vi "CIF_CIPC Channel Performance Test.vi"() -> ()   [LabVIEW 2021]
uses:
  <vilib>/Platform/TimedLoop/XDataNode/XDataNode.xnode
  <vilib>/Platform/TimedLoop/XDataNode/nitl_modes.ctl
  <vilib>/Platform/TimedLoop/XDataNode/XDNodeRunTimeDep.lvlib
  <vilib>/Platform/TimedLoop/XDataNode/wakeup.ctl
  <vilib>/Platform/TimedLoop/XDataNode/timing_clust.ctl
  CIFChannels/Typedef/Direction.ctl
  CIFChannels/CIFChannels.lvclass
  Double/CIF_CIPC_Chn_Double.lvclass
  826832b0-dd6f-429a-ad13-ef368b1fb745.vi
  9775e11d-bb16-4108-996d-a0b506d5c84d.vi
  c8328e1c-7f53-4066-9f95-efcf565d42f9.vi
  <vilib>/CIF Foundation/CIF CIPC/CIF_NI_CIPC.lvlib
  44731855-fec1-40f2-bc70-5f443bf403a0.vi
  ChannelCommon/typedef/New FIFO Instance Response.ctl
  ChannelCommon/ChannelCommon.lvlib
panel:
  in  "Stop":bool
  out "avg dbl channel":dbl
  out "max dbl channel":dbl
  out "avg raw channel":dbl
  out "max raw channel":dbl
  out "pass":bool
  out "error out":errorcluster
  # "This test should be run on RT.  It stresses the communications by constantly creating resource contraints with the low priority sender and the high priority loop. On Windows the priority of the loops cannot be set."
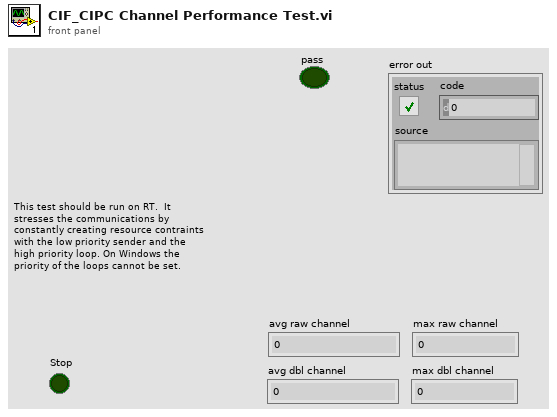
[diagram p1: front panel]
types:
  T1 = typedef "XDNodeRunTimeDep.lvlib/timing_clust.ctl" = cluster{"Expected End [f-1]":u64, "Actual End [f-1]":u64, "Finished Late? [f-1]":bool, "Expected End [i-1]":u64, "Actual End [i-1]":u64, "Finished Late? [i-1]":bool, "Expected Start [i]":u64, "Actual Start [i]":u64, "Expected Start [f]":u64, "Actual Start [f]":u64, "Source Name":string, "Structure Name":string, "Period":i64, "Deadline":i64, "Offset":i64, "Start":i64, "Priority":i32, "Timeout":i32, "Mode":T2, "Wakeup Reason":T3, "Error":errorcluster, "Source Type":string, "Secondary Source Type":string, "Global End Time":u64, "Global Start Time":u64, "Frame Duration":u64, "Iteration Duration":u64, "Assigned CPU":i32, "I/O Scan Engine Mode":u32}
  T2 = typedef "XDNodeRunTimeDep.lvlib/nitl_modes.ctl" = enum32{"No Change", "Process missed periods, maintain original phase", "Discard missed periods, maintain original phase", "Process missed periods, ignore original phase", "Discard missed periods, ignore original phase"}
  T3 = typedef "XDNodeRunTimeDep.lvlib/wakeup.ctl" = enum32{"Normal", "Aborted", "Asynchronous wakeup", "Timing source error", "Timed loop error", "Timeout"}
  T4 = typedef "ChannelCommon.lvlib/New FIFO Instance Response.ctl" = cluster{"Publisher":string, "Custom Data":u8[]}
  T5 = typedef "CIFChannels.lvclass/Direction.ctl" = enum16{"Publisher", "Subscriber"}
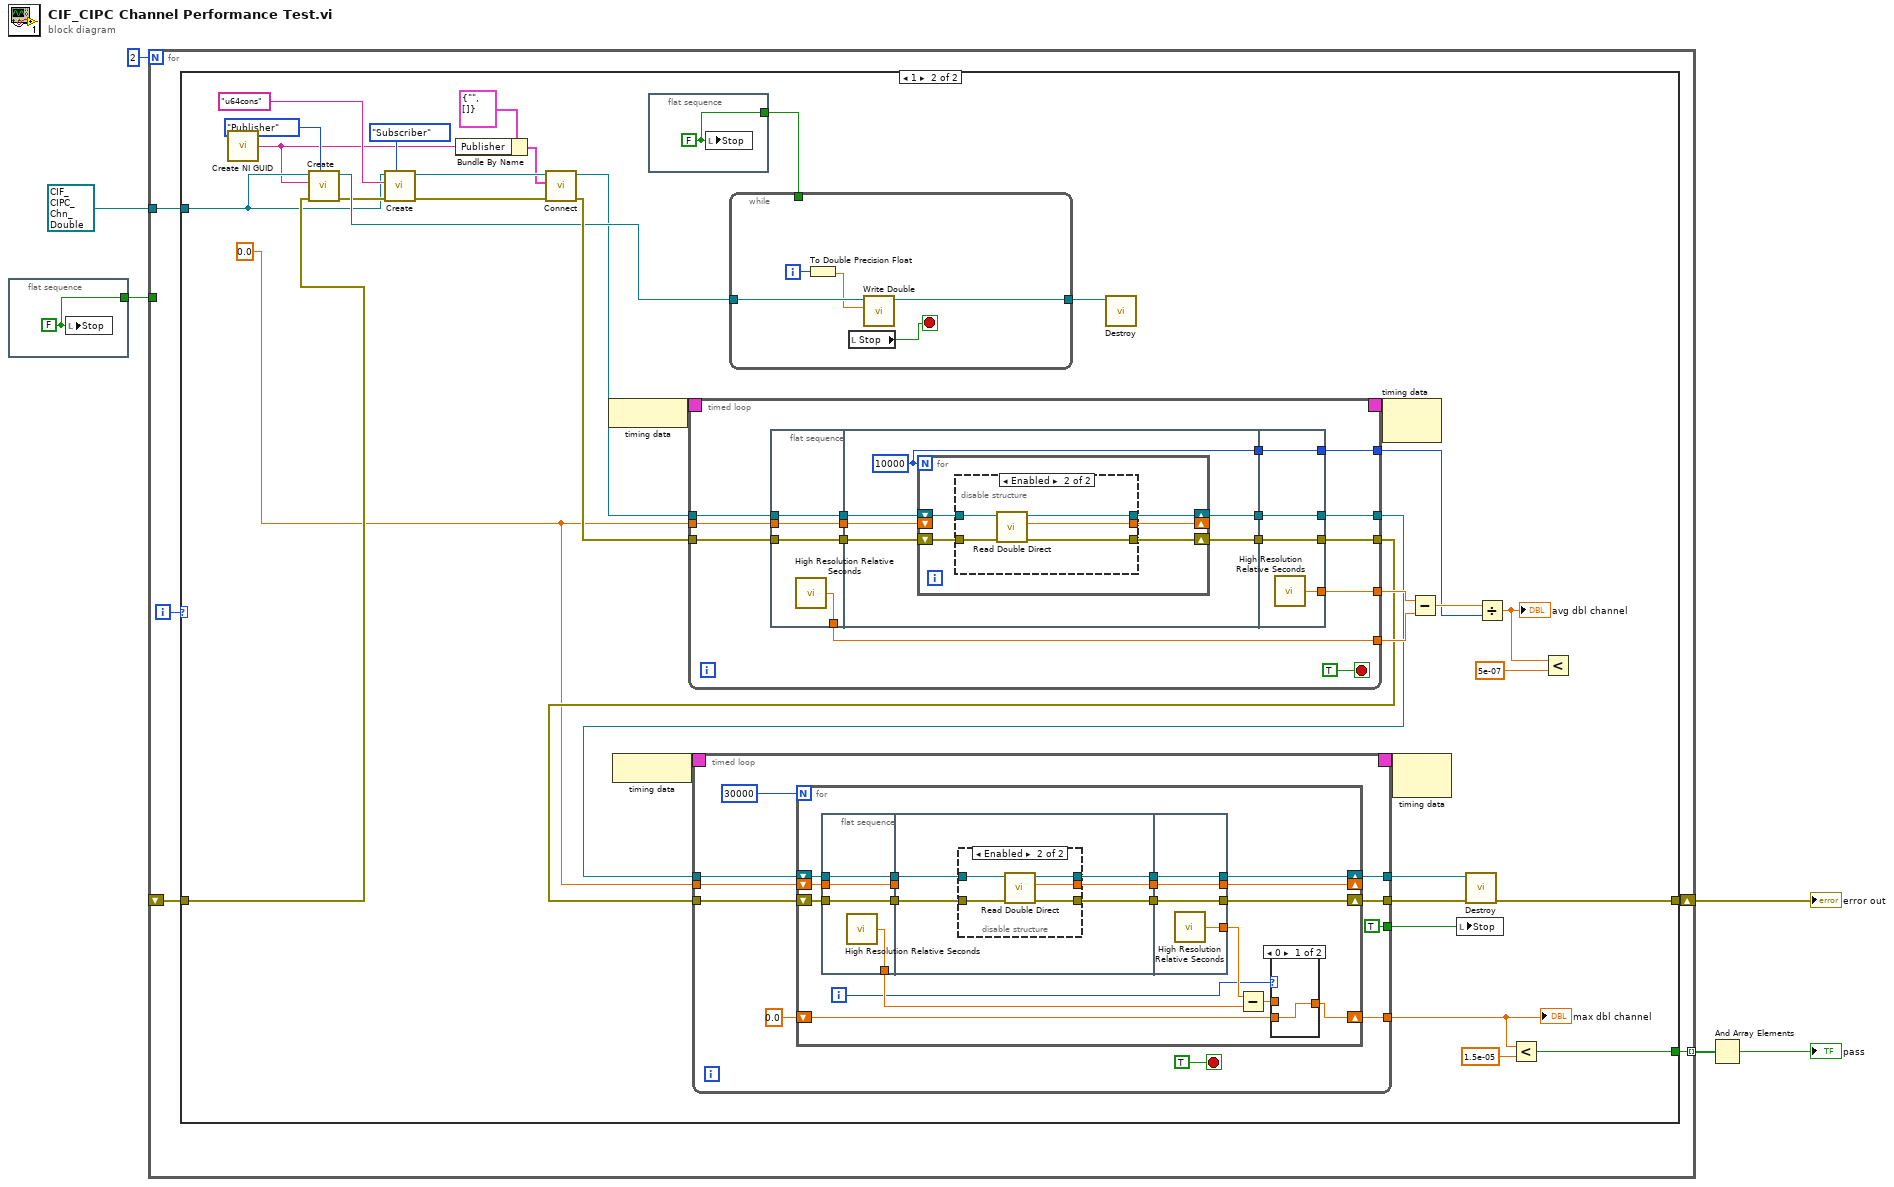
[diagram p0: block diagram]
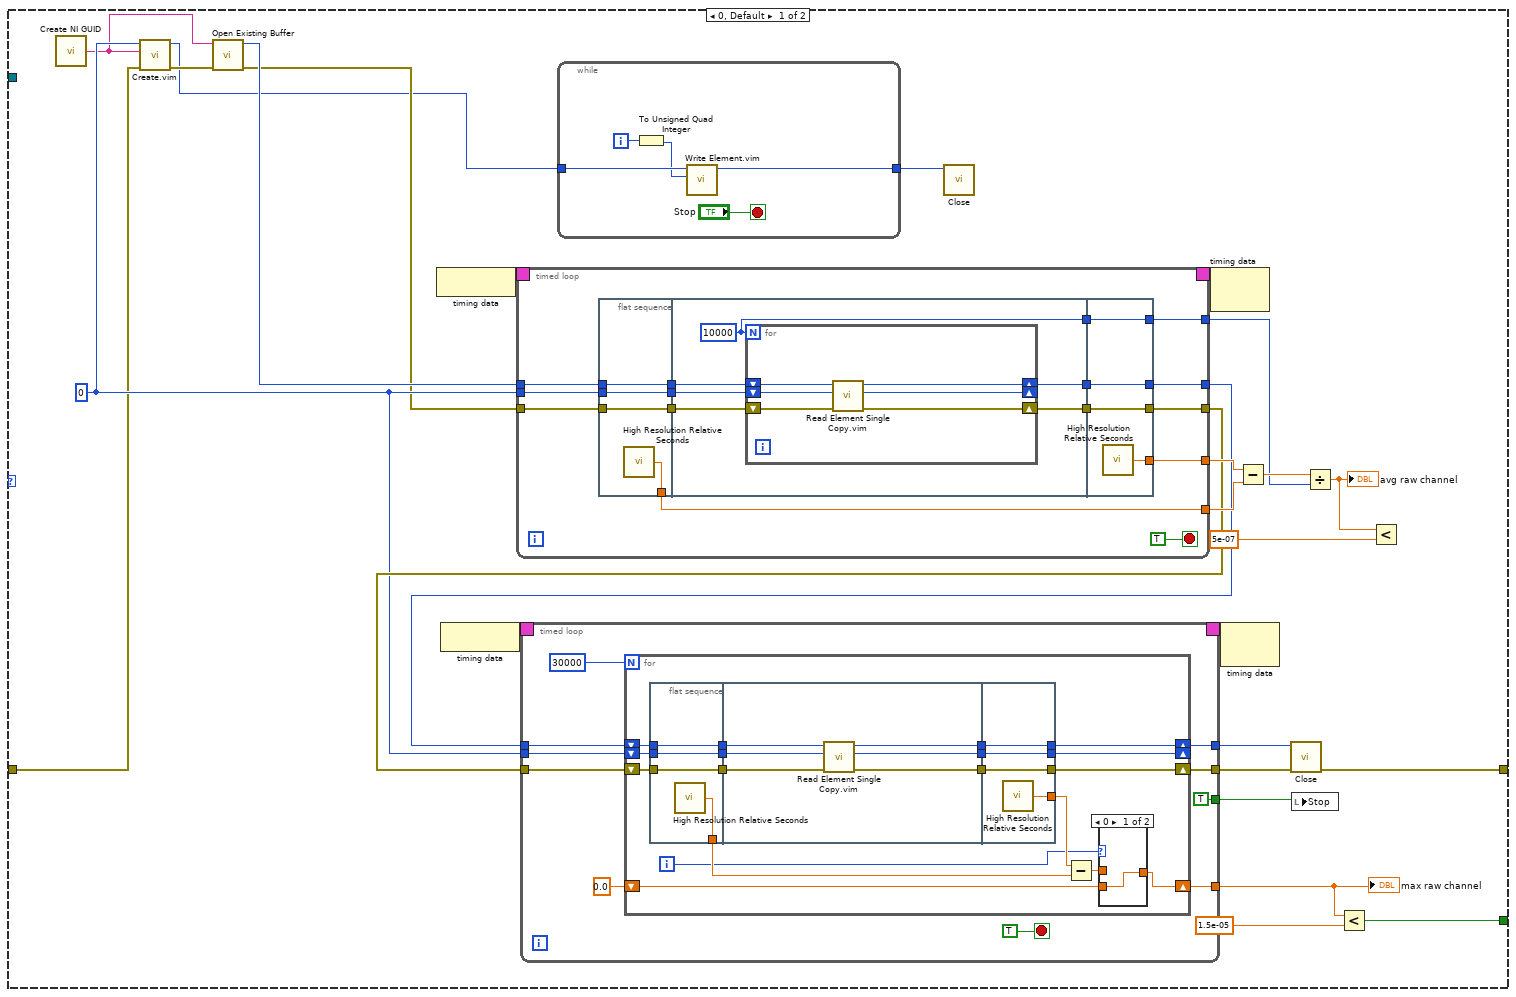
[diagram p2: hidden frame]
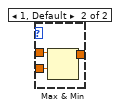
[diagram p3: hidden frame]
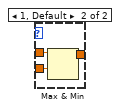
[diagram p4: hidden frame]
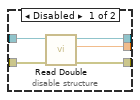
[diagram p5: hidden frame]
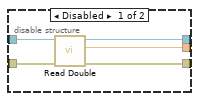
[diagram p6: hidden frame]
diagram:
  n1 = flat-sequence {
    tunnel: [w7] -> w1
    frame #0 {
      w7 = FALSE ("Stop")
      n2 = local write "Stop"(w7) -> ()
    }
  }
  n3 = for {
    N: 2 -> [_]
    tunnel: [w12] -> w4 mode=indexing
    shift-right: [w11] -> w6
    shift-left: _ -> [w9]
    tunnel: refnum<class "CIF_CIPC_Chn_Double.lvclass"> refnum ("CIF_CIPC_Chn_Double.lvclass") -> [w8]
    tunnel: w1 -> [_]
    i -> [w10]
    n4 = case shown="1" w10 {
      tunnel: [w25 w155] -> w12
      tunnel: [w15 w140] -> w11
      tunnel: w9 -> [w23 w153]
      tunnel: w8 -> [_ w142]
      frame 0, Default {
        w24 = u64 0
        n5 = call <vilib>:"Create NI GUID.vi"() -> ("NI GUID"=w22:string)
        n6 = call "Create.vim"("error in (no error)"=w23, "Name in"=w22, "Data Type"=w24) -> ("error out"=w21:errorcluster, "CIPC Reference"=w16:u64)  [unwired: 5 in, 2 out]
        n7 = call <vilib>:"Open Existing Buffer.vi"("error in (no error)"=w21, "buffer_name"=w22) -> ("error out"=w19:errorcluster, "CIPC Reference"=w20:u64)  [unwired: 8 in]
        n8 = node-c288() -> (w39:T1)
        n9 = node-c288() -> (w37:T1)
        n10 = timed-loop {
          timing: w39 -> [_]
          timing-out: [_] -> w38
          tunnel: w20 -> [w109]
          tunnel: w19 -> [w108]
          tunnel: [w104] -> w31
          tunnel: [w102] -> w30
          tunnel: [w100] -> w35
          tunnel: [w99] -> w34
          tunnel: [w98] -> w32
          tunnel: w24 -> [w96]
          stop <- TRUE stop-if-true
          n11 = flat-sequence {
            tunnel: w108 -> [w112]
            tunnel: w109 -> [w113]
            tunnel: [w113] -> w106
            tunnel: [w112] -> w105
            tunnel: [w111] -> w99
            tunnel: w96 -> [w110]
            tunnel: [w110] -> w95
            tunnel: w106 -> [w119]
            tunnel: w105 -> [w118]
            tunnel: [w117] -> w103
            tunnel: [w116] -> w101
            tunnel: [w115] -> w97
            tunnel: w95 -> [w114]
            tunnel: [w129] -> w104
            tunnel: w103 -> [w129]
            tunnel: [w128] -> w102
            tunnel: w101 -> [w128]
            tunnel: [w127] -> w100
            tunnel: [w126] -> w98
            tunnel: w97 -> [w126]
            frame #0 {
              n12 = call <vilib>:"High Resolution Relative Seconds.vi"() -> ("relative seconds"=w111:dbl)
            }
            frame #1 {
              w115 = 10000
              n13 = for {
                N: w115 -> [_]
                shift-right: [w120] -> w117
                shift-left: w119 -> [w125]
                shift-right: [w122] -> w116
                shift-left: w118 -> [w123]
                shift-right: [w121] -> _
                shift-left: w114 -> [w124]
                n14 = call "Read Element Single Copy.vim"("error in (no error)"=w123, "Data in"=w124, "CIPC Reference in"=w125) -> ("error out"=w122:errorcluster, "Data out"=w121:u64, "CIPC Reference out"=w120:u64)  [unwired: 4 in, 2 out]
              }
            }
            frame #2 {
              n15 = call <vilib>:"High Resolution Relative Seconds.vi"() -> ("relative seconds"=w127:dbl)
            }
          }
        }
        n16 = timed-loop {
          timing: w37 -> [_]
          timing-out: [_] -> w36
          tunnel: w31 -> [w54]
          tunnel: w30 -> [w53]
          tunnel: [w51] -> w18
          tunnel: [w50] -> w17
          tunnel: w24 -> [w49]
          tunnel: [w46] -> w27
          tunnel: [TRUE ("Stop")] -> w14
          stop <- TRUE stop-if-true
          n17 = for {
            N: 30000 -> [_]
            shift-right: [w66] -> w51
            shift-left: w54 -> [w68]
            shift-right: [w65] -> w50
            shift-left: w53 -> [w67]
            shift-right: [w59] -> w46
            shift-left: 0.0 -> [w60]
            shift-right: [w58] -> _
            shift-left: w49 -> [w64]
            i -> [w56]
            n18 = flat-sequence {
              tunnel: w67 -> [w79]
              tunnel: w68 -> [w80]
              tunnel: [w80] -> w72
              tunnel: [w79] -> w71
              tunnel: [w78] -> w62
              tunnel: w64 -> [w77]
              tunnel: [w77] -> w70
              tunnel: w72 -> [w86]
              tunnel: w71 -> [w84]
              tunnel: [w81] -> w69
              tunnel: w70 -> [w85]
              tunnel: [w82] -> w57
              tunnel: [w83] -> w55
              tunnel: [w90] -> w66
              tunnel: w69 -> [w90]
              tunnel: [w89] -> w65
              tunnel: [w88] -> w63
              tunnel: [w87] -> w58
              tunnel: w57 -> [w87]
              tunnel: w55 -> [w89]
              frame #0 {
                n19 = call <vilib>:"High Resolution Relative Seconds.vi"() -> ("relative seconds"=w78:dbl)
              }
              frame #1 {
                n20 = call "Read Element Single Copy.vim"("error in (no error)"=w84, "Data in"=w85, "CIPC Reference in"=w86) -> ("error out"=w83:errorcluster, "Data out"=w82:u64, "CIPC Reference out"=w81:u64)  [unwired: 4 in, 2 out]
              }
              frame #2 {
                n21 = call <vilib>:"High Resolution Relative Seconds.vi"() -> ("relative seconds"=w88:dbl)
              }
            }
            n22 = Subtract(x=w63, y=w62) -> (x-y=w61:dbl)
            n23 = case shown="0" w56 {
              tunnel: w61 -> [_ w76]
              tunnel: w60 -> [w73 w75]
              tunnel: [w73 w74] -> w59
              frame 0 {
              }
              frame 1, Default {
                n24 = Max & Min(x=w76, y=w75) -> (max(x,y)=w74:dbl)  [unwired: 1 out]
              }
            }
          }
        }
        "max raw channel" <- w27
        n25 = while {
          tunnel: w16 -> [w43]
          tunnel: [w40] -> w13
          i -> [w44]
          stop <- "Stop" stop-if-true
          n26 = To Unsigned Quad Integer(1:w44) -> (0:w42:u64)
          n27 = call "Write Element.vim"("Data in"=w42, "CIPC Reference in"=w43) -> ("CIPC Reference out"=w40:u64)  [unwired: 6 in, 3 out]
        }
        n28 = call <vilib>:"Close.vi"("CIPC Reference"=w13) -> ()  [unwired: 10 in, 1 out]
        n29 = node-c288(w38) -> ()  [unwired: 1 out]
        n30 = node-c288(w36) -> ()  [unwired: 1 out]
        n31 = Subtract(x=w35, y=w34) -> (x-y=w33:dbl)
        n32 = call <vilib>:"Close.vi"("error in (no error)"=w17, "CIPC Reference"=w18) -> ("error out"=w15:errorcluster)  [unwired: 9 in]
        n33 = local write "Stop"(w14) -> ()
        n34 = Divide(x=w33, y=w32) -> (x/y=w29:dbl)
        "avg raw channel" <- w29
        n35 = Less?(x=w27, y=1.5e-05) -> (x < y?=w25:bool)
        n36 = Less?(x=w29, y=5e-07) -> ()  [unwired: 1 out]
      }
      frame 1 {
        w149 = 0.0
        n37 = call <vilib>:"Create NI GUID.vi"() -> ("NI GUID"=w135:string)
        n38 = call-dynamic "Create.vi"("Direction"=Direction."Publisher", "error in (no error)"=w153, "Name"=w135, "CIFTag in"=w142) -> ("error out"=w148:errorcluster, "CIFTag out"=w150:refnum<class "CIF_CIPC_Chn_Double.lvclass">)  [unwired: 6 in]
        n39 = call-dynamic "Create.vi"("Direction"=Direction."Subscriber", "error in (no error)"=w148, "Name"="u64cons" ("Channel Name"), "CIFTag in"=w142) -> ("error out"=w146:errorcluster, "CIFTag out"=w145:refnum<class "CIF_CIPC_Chn_Double.lvclass">)  [unwired: 6 in]
        n40 = Bundle By Name(cluster=T4 {"Publisher"="", "Custom Data"=[]} ("Connection"), "Publisher"=w135) -> (w134:T4)
        n41 = call-dynamic "Connect.vi"("error in (no error)"=w146, "Connection"=w134, "CIFTag in"=w145) -> ("error out"=w154:errorcluster, "CIFTag out"=w144:refnum<class "CIF_CIPC_Chn_Double.lvclass">)  [unwired: 7 in]
        n42 = node-c288() -> (w169:T1)
        n43 = node-c288() -> (w167:T1)
        n44 = flat-sequence {
          tunnel: [w170] -> w138
          frame #0 {
            w170 = FALSE ("Stop")
            n45 = local write "Stop"(w170) -> ()
          }
        }
        n46 = timed-loop {
          timing: w169 -> [_]
          timing-out: [_] -> w168
          tunnel: w144 -> [w249]
          tunnel: w154 -> [w248]
          tunnel: [w244] -> w161
          tunnel: [w242] -> w160
          tunnel: [w240] -> w165
          tunnel: [w239] -> w164
          tunnel: [w238] -> w162
          tunnel: w149 -> [w236]
          stop <- TRUE stop-if-true
          n47 = flat-sequence {
            tunnel: w248 -> [w252]
            tunnel: w249 -> [w253]
            tunnel: [w253] -> w246
            tunnel: [w252] -> w245
            tunnel: [w251] -> w239
            tunnel: w236 -> [w250]
            tunnel: [w250] -> w235
            tunnel: w246 -> [w259]
            tunnel: w245 -> [w258]
            tunnel: [w257] -> w243
            tunnel: [w256] -> w241
            tunnel: [w255] -> w237
            tunnel: w235 -> [w254]
            tunnel: [w278] -> w244
            tunnel: w243 -> [w278]
            tunnel: [w277] -> w242
            tunnel: w241 -> [w277]
            tunnel: [w276] -> w240
            tunnel: [w275] -> w238
            tunnel: w237 -> [w275]
            frame #0 {
              n48 = call <vilib>:"High Resolution Relative Seconds.vi"() -> ("relative seconds"=w251:dbl)
            }
            frame #1 {
              w255 = 10000
              n49 = for {
                N: w255 -> [_]
                shift-right: [w262] -> w257
                shift-left: w259 -> [w264]
                shift-right: [w261] -> w256
                shift-left: w258 -> [w260]
                shift-right: [w263] -> _
                shift-left: w254 -> [_]
                n50 = disable-structure shown="Enabled" {
                  disable-tunnel: w264 -> [w269 w274]
                  disable-tunnel: [w268 w270] -> w263
                  disable-tunnel: [w267 w271] -> w262
                  disable-tunnel: [w266 w272] -> w261
                  disable-tunnel: w260 -> [w265 w273]
                  frame Disabled {
                    n51 = call-dynamic "Read Double.vi"("error in (no error)"=w265, "CIFTag in"=w269) -> ("error out"=w266:errorcluster, "Data"=w268:dbl, "CIFTag out"=w267:refnum<class "CIF_CIPC_Chn_Double.lvclass">)  [unwired: 6 in, 1 out]
                  }
                  frame Enabled {
                    n52 = call "Read Double Direct.vi"("error in (no error)"=w273, "CIFTag in"=w274) -> ("error out"=w272:errorcluster, "Data"=w270:dbl, "CIFTag out"=w271:refnum<class "CIF_CIPC_Chn_Double.lvclass">)  [unwired: 6 in, 1 out]
                  }
                }
              }
            }
            frame #2 {
              n53 = call <vilib>:"High Resolution Relative Seconds.vi"() -> ("relative seconds"=w276:dbl)
            }
          }
        }
        n54 = timed-loop {
          timing: w167 -> [_]
          timing-out: [_] -> w166
          tunnel: w161 -> [w185]
          tunnel: w160 -> [w184]
          tunnel: [w182] -> w151
          tunnel: [w181] -> w152
          tunnel: w149 -> [w180]
          tunnel: [w177] -> w157
          tunnel: [TRUE ("Stop")] -> w137
          stop <- TRUE stop-if-true
          n55 = for {
            N: 30000 -> [_]
            shift-right: [w197] -> w182
            shift-left: w185 -> [w199]
            shift-right: [w196] -> w181
            shift-left: w184 -> [w198]
            shift-right: [w190] -> w177
            shift-left: 0.0 -> [w191]
            shift-right: [w189] -> _
            shift-left: w180 -> [w195]
            i -> [w187]
            n56 = flat-sequence {
              tunnel: w198 -> [w210]
              tunnel: w199 -> [w211]
              tunnel: [w211] -> w203
              tunnel: [w210] -> w202
              tunnel: [w209] -> w193
              tunnel: w195 -> [w208]
              tunnel: [w208] -> w201
              tunnel: w203 -> [w216]
              tunnel: w202 -> [w213]
              tunnel: [w215] -> w200
              tunnel: w201 -> [_]
              tunnel: [w214] -> w188
              tunnel: [w212] -> w186
              tunnel: [w230] -> w197
              tunnel: w200 -> [w230]
              tunnel: [w229] -> w196
              tunnel: [w228] -> w194
              tunnel: [w227] -> w189
              tunnel: w188 -> [w227]
              tunnel: w186 -> [w229]
              frame #0 {
                n57 = call <vilib>:"High Resolution Relative Seconds.vi"() -> ("relative seconds"=w209:dbl)
              }
              frame #1 {
                n58 = disable-structure shown="Enabled" {
                  disable-tunnel: w216 -> [w221 w226]
                  disable-tunnel: [w220 w222] -> w215
                  disable-tunnel: [w219 w223] -> w214
                  disable-tunnel: w213 -> [w218 w225]
                  disable-tunnel: [w217 w224] -> w212
                  frame Disabled {
                    n59 = call-dynamic "Read Double.vi"("error in (no error)"=w218, "CIFTag in"=w221) -> ("error out"=w217:errorcluster, "Data"=w219:dbl, "CIFTag out"=w220:refnum<class "CIF_CIPC_Chn_Double.lvclass">)  [unwired: 6 in, 1 out]
                  }
                  frame Enabled {
                    n60 = call "Read Double Direct.vi"("error in (no error)"=w225, "CIFTag in"=w226) -> ("error out"=w224:errorcluster, "Data"=w223:dbl, "CIFTag out"=w222:refnum<class "CIF_CIPC_Chn_Double.lvclass">)  [unwired: 6 in, 1 out]
                  }
                }
              }
              frame #2 {
                n61 = call <vilib>:"High Resolution Relative Seconds.vi"() -> ("relative seconds"=w228:dbl)
              }
            }
            n62 = Subtract(x=w194, y=w193) -> (x-y=w192:dbl)
            n63 = case shown="0" w187 {
              tunnel: w192 -> [_ w207]
              tunnel: w191 -> [w204 w206]
              tunnel: [w204 w205] -> w190
              frame 0 {
              }
              frame 1, Default {
                n64 = Max & Min(x=w207, y=w206) -> (max(x,y)=w205:dbl)  [unwired: 1 out]
              }
            }
          }
        }
        "max dbl channel" <- w157
        n65 = while {
          tunnel: w150 -> [w174]
          tunnel: [w172] -> w139
          tunnel: w138 -> [_]
          i -> [w175]
          stop <- w171 stop-if-true
          n66 = To Double Precision Float(number=w175) -> (double precision float=w173:dbl)
          n67 = local read "Stop"() -> (w171:bool)
          n68 = call-dynamic "Write Double.vi"("Data"=w173, "CIFTag in"=w174) -> ("CIFTag out"=w172:refnum<class "CIF_CIPC_Chn_Double.lvclass">)  [unwired: 7 in, 2 out]
        }
        n69 = call-dynamic "Destroy.vi"("CIFTag in"=w139) -> ()  [unwired: 9 in, 2 out]
        n70 = node-c288(w168) -> ()  [unwired: 1 out]
        n71 = node-c288(w166) -> ()  [unwired: 1 out]
        n72 = Subtract(x=w165, y=w164) -> (x-y=w163:dbl)
        n73 = local write "Stop"(w137) -> ()
        n74 = call-dynamic "Destroy.vi"("error in (no error)"=w152, "CIFTag in"=w151) -> ("error out"=w140:errorcluster)  [unwired: 8 in, 1 out]
        n75 = Divide(x=w163, y=w162) -> (x/y=w159:dbl)
        "avg dbl channel" <- w159
        n76 = Less?(x=w157, y=1.5e-05) -> (x < y?=w155:bool)
        n77 = Less?(x=w159, y=5e-07) -> ()  [unwired: 1 out]
      }
    }
  }
  "error out" <- w6
  n78 = And Array Elements(Boolean array=w4) -> (logical AND=→"pass":bool)
